vi "Setup Registry.vi"() -> ()   [LabVIEW 2012]
uses:
  <vilib>/registry/registry.llb/Registry RtKey.ctl
  <vilib>/registry/registry.llb/Write Registry Value Simple STR.vi
panel:
  out "Application:Command Line Arguments":string[](array[string])
  in  "Run":bool
  in  "Remove Keys":bool
  in  "Installed Directory":path=path "C:/Program Files (x86)/Version Checker/VIVersionChecker.exe"
  in  "Classes":string[](array[string])=["LabVIEWInstrument", "LabVIEWProject", "LabVIEWClass", "LabVIEWLibrary", "LabVIEWPacked Library", "LabVIEWControl", "LabVIEWControlTemplate", "LabVIEWInstrumentTemplate", "LabVIEWXControl"]
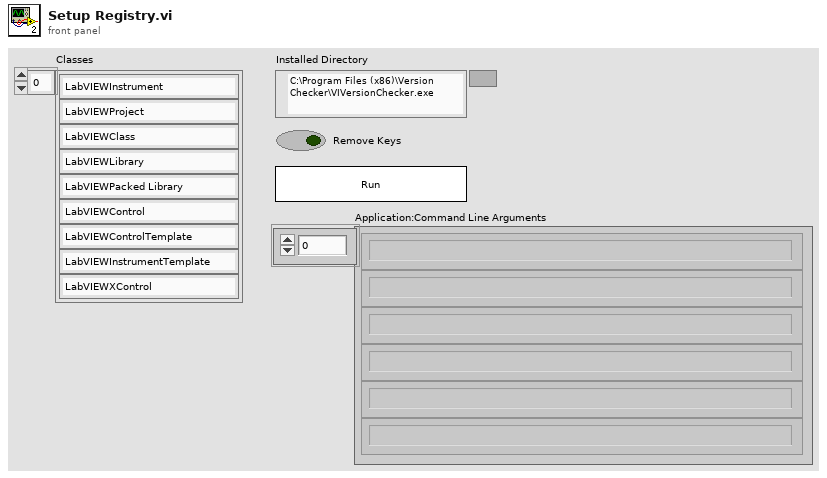
[diagram p1: front panel]
types:
  T1 = typedef "Registry RtKey.ctl" = enum32{"HKEY_CLASSES_ROOT", "HKEY_CURRENT_USER", "HKEY_LOCAL_MACHINE", "HKEY_USERS", "HKEY_PERFORMANCE_DATA", "HKEY_CURRENT_CONFIG", "HKEY_DYN_DATA"}
  T2 = typedef "Registry refnum.ctl" = refnum<k1>
  T3 = enum32{"invalid app kind", "Development System", "Run Time System", "Student Edition", "Embedded LabVIEW", "Evaluation", "Custom"}
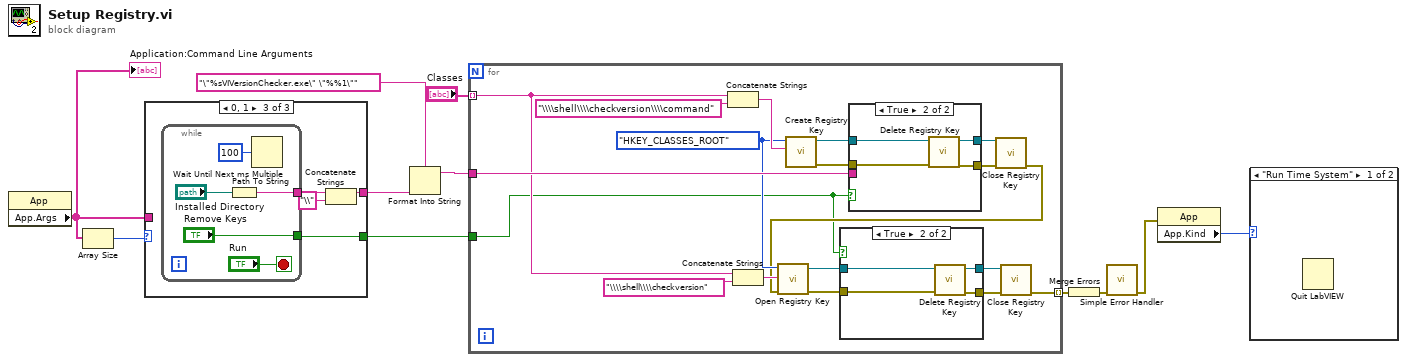
[diagram p0: block diagram]
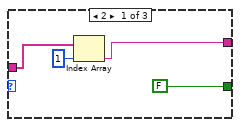
[diagram p3: hidden frame]
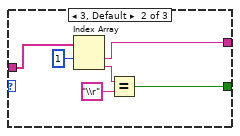
[diagram p4: hidden frame]
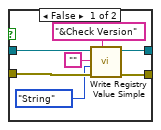
[diagram p5: hidden frame]
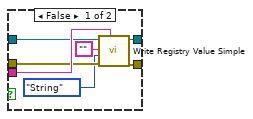
[diagram p6: hidden frame]
diagram:
  n1 = property class="App"() -> ("App.Args"=w3:string[])  [unwired: 2 in, 2 out]
  "Application:Command Line Arguments" <- w3
  n2 = Array Size(array=w3) -> (size(s)=w4:i32)
  n3 = case shown="0, 1" w4 {
    tunnel: [w13 w19 w23] -> w10
    tunnel: [FALSE ("Remove Keys") w16 w24] -> w7
    tunnel: w3 -> [w15 w21 _]
    frame 2 {
      n4 = Index Array(array=w15, index=1) -> (element=w13:string)
    }
    frame 3, Default {
      n5 = Index Array(array=w21, index #1=1 ("index")) -> (element #1=w19:string, element #2=w18:string)  [unwired: 1 in]
      n6 = Equal?(x=w18, y="\\r") -> (x = y?=w16:bool)
    }
    frame 0, 1 {
      n7 = while {
        tunnel: [w29] -> w25
        tunnel: ["Remove Keys"] -> w24
        stop <- "Run" stop-if-true
        n8 = Path To String(path="Installed Directory") -> (string=w29:string)
        n9 = Wait Until Next ms Multiple(millisecond multiple=u32 100) -> ()  [unwired: 1 out]
      }
      n10 = Concatenate Strings(w25, "\\" ("string")) -> (w23:string)
    }
  }
  n11 = Format Into String(format string="\"%sVIVersionChecker.exe\" \"%%1\"", w10) -> (resulting string=w8:string)  [unwired: 2 in, 1 out]
  n12 = for {
    tunnel: "Classes" -> [w47] mode=indexing
    tunnel: w8 -> [w48]
    tunnel: w7 -> [w32]
    tunnel: [w31] -> w6 mode=indexing
    w40 = Registry_RtKey."HKEY_CLASSES_ROOT" ("root key (HKEY_LOCAL_MACHINE)")
    n13 = Concatenate Strings(w47, "\\\\shell\\\\checkversion\\\\command" ("string")) -> (w45:string)
    n14 = Concatenate Strings(w47, "\\\\shell\\\\checkversion" ("string")) -> (w38:string)
    n15 = call <vilib>:"Create Registry Key.vi"("subkey"=w45, "root key (HKEY_LOCAL_MACHINE)"=w40) -> ("error out"=w43:errorcluster, "refnum out"=w44:T2)  [unwired: 7 in, 1 out]
    n16 = case shown="True" w32 {
      tunnel: w48 -> [w66 _]
      tunnel: w44 -> [w65 w67]
      tunnel: w43 -> [w64 w68]
      tunnel: [w63 w69] -> w42
      tunnel: [w62 w70] -> w41
      frame False {
        n17 = call-poly <vilib>:"Write Registry Value Simple.vi"("String/Binary data"=w66, "error in (no error)"=w64, "simple data type"=enum16{"String", "Binary", "DWORD"}."String", "value"="", "refnum"=w65) -> ("error out"=w63:errorcluster, "refnum out"=w62:T2)  [unwired: 3 in]
      }
      frame True {
        n18 = call <vilib>:"Delete Registry Key.vi"("error in (no error)"=w68, "refnum"=w67) -> ("error out"=w69:errorcluster, "refnum out"=w70:T2)  [unwired: 8 in]
      }
    }
    n19 = call <vilib>:"Close Registry Key.vi"("error in (no error)"=w42, "refnum"=w41) -> ("error out"=w33:errorcluster)  [unwired: 5 in]
    n20 = call <vilib>:"Open Registry Key.vi"("error in (no error)"=w33, "subkey"=w38, "root key (HKEY_LOCAL_MACHINE)"=w40) -> ("error out"=w37:errorcluster, "refnum out"=w34:T2)  [unwired: 7 in]
    n21 = case shown="True" w32 {
      tunnel: w37 -> [w54 w56]
      tunnel: [w53 w59] -> w36
      tunnel: [w52 w58] -> w35
      tunnel: w34 -> [w51 w57]
      frame False {
        n22 = call-poly <vilib>:"Write Registry Value Simple.vi"("String/Binary data"="&Check Version", "error in (no error)"=w54, "simple data type"=enum16{"String", "Binary", "DWORD"}."String", "value"="", "refnum"=w51) -> ("error out"=w53:errorcluster, "refnum out"=w52:T2)  [unwired: 3 in]
      }
      frame True {
        n23 = call <vilib>:"Delete Registry Key.vi"("error in (no error)"=w56, "refnum"=w57) -> ("error out"=w59:errorcluster, "refnum out"=w58:T2)  [unwired: 8 in]
      }
    }
    n24 = call <vilib>:"Close Registry Key.vi"("error in (no error)"=w36, "refnum"=w35) -> ("error out"=w31:errorcluster)  [unwired: 5 in]
  }
  n25 = Merge Errors(w6) -> (w5:errorcluster)
  n26 = call <vilib>:"Simple Error Handler.vi"("error in (no error)"=w5) -> ("error out"=w1:errorcluster)  [unwired: 4 in, 4 out]
  n27 = property class="App"(error in=w1) -> ("App.Kind"=w2:T3)  [unwired: 1 in, 2 out]
  n28 = case shown="\"Run Time System\"" w2 {
    frame "Run Time System" {
      n29 = Quit LabVIEW() -> ()  [unwired: 1 in]
    }
    frame "Development System", Default {
    }
  }
